vi "apply key value pairs.vi"(8 "error in":errorcluster, 9 "values":string[](array[string]), 10 "keys":string[](array[string]), 11 "fixed channel runtime in":refnum<class "Custom Temperature Controller runtime.lvclass">) -> (0 "error out":errorcluster, 3 "fixed channel runtime out":refnum<class "Custom Temperature Controller runtime.lvclass">)   [LabVIEW 2021, in "Custom Temperature Controller runtime.lvclass"]
uses:
  Custom Temperature Controller runtime.lvclass
  Custom Temperature Controller runtime.lvclass/Custom Temperature Controller runtime.ctl
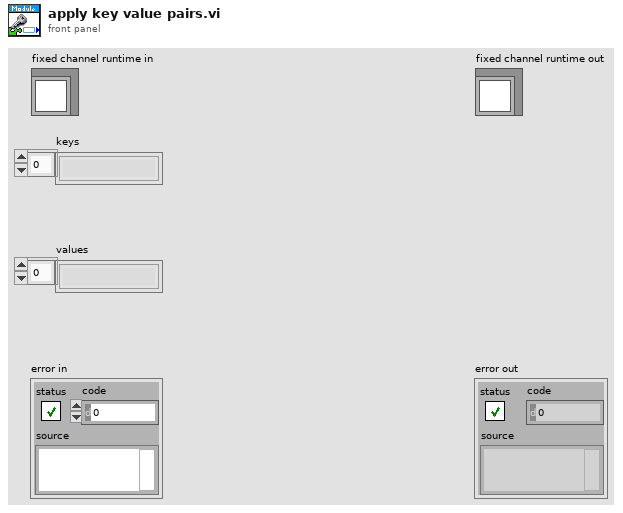
[diagram p1: front panel]
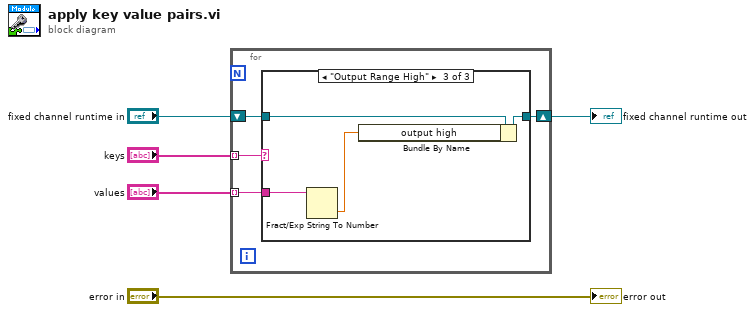
[diagram p0: block diagram]
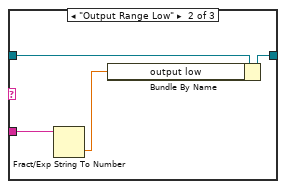
[diagram p3: hidden frame]
diagram:
  n1 = for {
    shift-right: [w6] -> w4
    shift-left: "fixed channel runtime in" -> [w7]
    tunnel: "keys" -> [w9] mode=indexing
    tunnel: "values" -> [w8] mode=indexing
    n2 = case shown="\"Output Range High\"" w9 {
      tunnel: w8 -> [_ w14 w18]
      tunnel: w7 -> [w10 w13 w17]
      tunnel: [w10 w12 w16] -> w6
      frame Default {
      }
      frame "Output Range Low" {
        n3 = Fract/Exp String To Number(string=w14) -> (number=w11:dbl)  [unwired: 3 in, 1 out]
        n4 = Bundle By Name(cluster=w13, "output low"=w11) -> (w12:refnum<class "Custom Temperature Controller runtime.lvclass">)
      }
      frame "Output Range High" {
        n5 = Fract/Exp String To Number(string=w18) -> (number=w15:dbl)  [unwired: 3 in, 1 out]
        n6 = Bundle By Name(cluster=w17, "output high"=w15) -> (w16:refnum<class "Custom Temperature Controller runtime.lvclass">)
      }
    }
  }
  "fixed channel runtime out" <- w4
  "error out" <- "error in"
